vi "Create Directed Graph Map.vi"(8 "error in (no error)":errorcluster, 9 "heuristic function":u16(ring) items=["Euclidean Distance", "Manhattan Distance"], 11 "nodes":cluster{"name":string, "coordinates":dbl[]}[](array[cluster])) -> (0 "error out":errorcluster, 3 "map reference out":refnum<data-value>)   [LabVIEW 2017, in "NI_Robotics_DirectedGraphWorldMap.lvclass"]
doc: "Generates a map of the robot environment that consists of irregularly spaced points, or <B>nodes</B>."
uses:
  <vilib>/robotics/Navigation/shared/WorldMap/DirectedGraphWorldMap/NI_Robotics_DirectedGraphWorldMap.lvclass
  <vilib>/robotics/Navigation/shared/WorldMap/DirectedGraphWorldMap/NI_Robotics_DirectedGraphWorldMap.lvclass/NI_Robotics_DirectedGraphWorldMap.ctl
  <vilib>/robotics/Navigation/shared/MapNode/DirectedGraphMapNode/NI_Robotics_DirectedGraphMapNode.lvclass
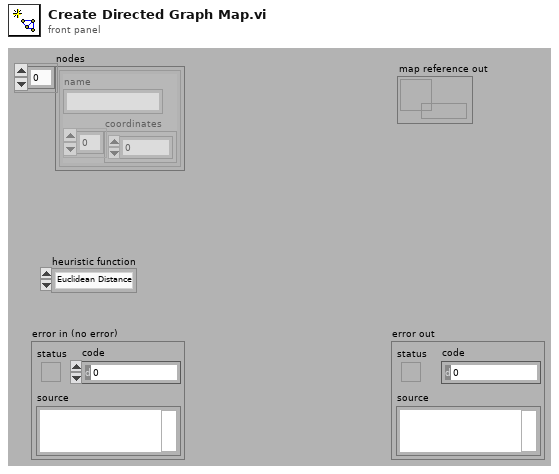
[diagram p1: front panel]
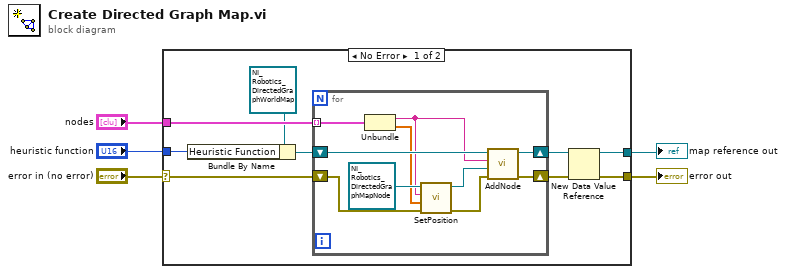
[diagram p0: block diagram]
diagram:
  n1 = case shown="No Error" "error in (no error)" {
    selector: "error in (no error)" -> [w11 w25]
    tunnel: "heuristic function" -> [w14 _]
    tunnel: [w6 _] -> w2
    tunnel: "nodes" -> [w13 _]
    tunnel: [w7 w25] -> w1
    frame No Error {
      n2 = Bundle By Name(cluster=refnum<class "NI_Robotics_DirectedGraphWorldMap.lvclass"> refnum ("DirectedGraphWorldMap.lvclass"), "Heuristic Function"=w14) -> (w12:refnum<class "NI_Robotics_DirectedGraphWorldMap.lvclass">)
      n3 = for {
        tunnel: w13 -> [w24] mode=indexing
        shift-right: [w18] -> w8
        shift-left: w11 -> [w22]
        shift-right: [w17] -> w9
        shift-left: w12 -> [w20]
        n4 = Unbundle(w24) -> ("name"=w15:string, "coordinates"=w16:dbl[])
        n5 = call-dynamic "SetPosition.vi"("error in (no error)"=w22, "coordinates"=w16, "name"=w15, "DirectedGraphMapNode in"=refnum<class "NI_Robotics_DirectedGraphMapNode.lvclass"> refnum ("DirectedGraphMapNode.lvclass")) -> ("error out"=w21:errorcluster, "DirectedGraphMapNode out"=w19:refnum<class "NI_Robotics_DirectedGraphMapNode.lvclass">)  [unwired: 6 in]
        n6 = call-dynamic "AddNode.vi"("error in (no error)"=w21, "DirectedGraphMapNode.lvclass"=w19, "Name"=w15, "DirectedGraphWorldMap in"=w20) -> ("error out"=w18:errorcluster, "DirectedGraphWorldMap out"=w17:refnum<class "NI_Robotics_DirectedGraphWorldMap.lvclass">)  [unwired: 5 in, 1 out]
      }
      n7 = New Data Value Reference(data value=w9, error in=w8) -> (data value reference=w6:refnum<data-value>, error out=w7:errorcluster)
    }
    frame Error {
    }
  }
  "map reference out" <- w2
  "error out" <- w1
